vi "Database - Read Entry.vi"(0 "reference in":refnum<class "Database_UUT.lvclass">, 4 "Part Number":string, 5 "error in (no error)":errorcluster) -> (9 "Data Waveform":waveform(dbl), 11 "Property Names":string[](array[string]), 13 "Property Values":variant[](array[variant]), 14 "reference out":refnum<class "Database_UUT.lvclass">, 17 "Channel Name":string, 18 "Part Number OUT":string, 19 "error out":errorcluster)   [LabVIEW 2017, in "Database_UUT.lvclass"]
uses:
  Database_UUT.lvclass
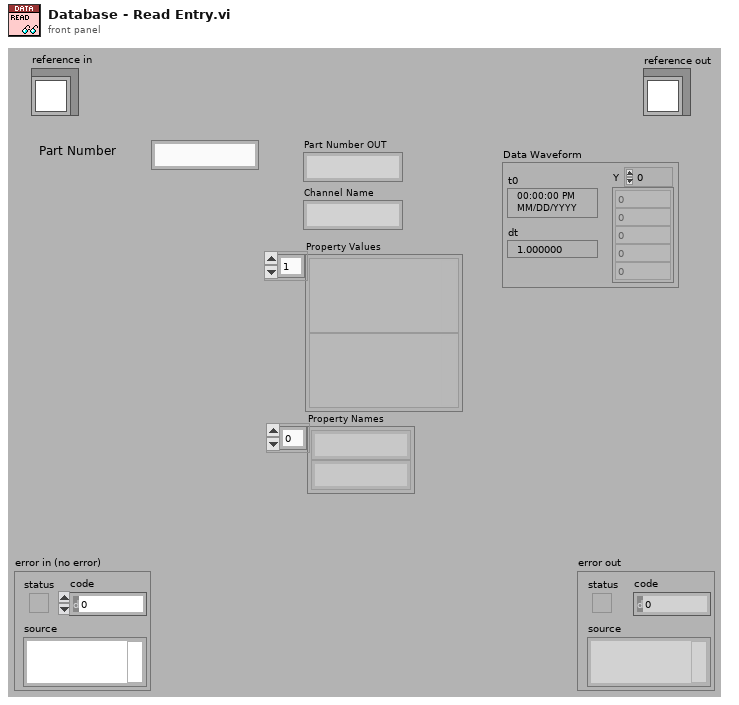
[diagram p1: front panel]
types:
  T1 = enum16{"open", "open or create", "create or replace", "create", "open (read-only)"}
  T2 = typedef "Database_UUT.lvclass/ObjectAttributes.ctl" = cluster{"Filepath to Database":path}
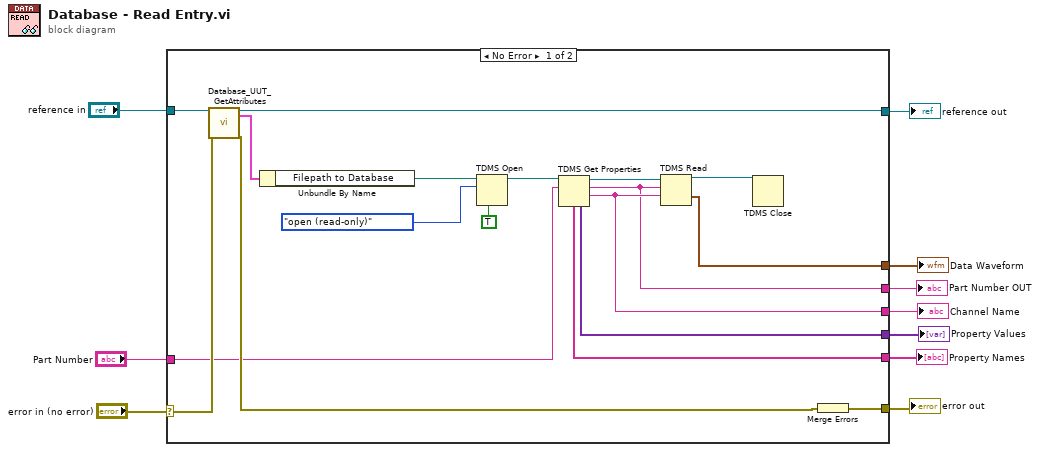
[diagram p0: block diagram]
diagram:
  n1 = case shown="No Error" "error in (no error)" {
    selector: "error in (no error)" -> [w27 w30]
    tunnel: [w23 w30] -> w9
    tunnel: [w25 w29] -> w7
    tunnel: "reference in" -> [w28 w29]
    tunnel: "Part Number" -> [w19 _]
    tunnel: [w12 _] -> w5
    tunnel: [w18 _] -> w4
    tunnel: [w16 _] -> w3
    tunnel: [w14 _] -> w2
    tunnel: [w13 _] -> w1
    frame No Error {
      n2 = call "Database_UUT_GetAttributes.vi"("reference in"=w28, "error in (no error)"=w27) -> ("reference out"=w25:refnum<class "Database_UUT.lvclass">, "Data"=w26:T2, "error out"=w22:errorcluster)  [unwired: 14 in, 1 out]
      n3 = Unbundle By Name(w26) -> ("Filepath to Database"=w21:path)
      n4 = TDMS Open(6:TRUE ("enable asynchronous? (T)"), 10:T1."open (read-only)" ("operation (0:open)"), 11:w21) -> (3:w17:refnum<k34>)  [unwired: 4 in, 1 out]
      n5 = TDMS Get Properties(10:w19, 11:w17) -> (1:w14:string, 2:w12:string, 3:w15:refnum<k34>, 4:w16:variant[], 6:w18:string[])  [unwired: 4 in, 1 out]
      n6 = TDMS Read(0:w15, 5:w12, 7:w14) -> (4:w11:refnum<k34>, 10:w13:waveform(dbl))  [unwired: 5 in, 4 out]
      n7 = TDMS Close(11:w11) -> ()  [unwired: 1 in, 2 out]
      n8 = Merge Errors(w22) -> (w23:errorcluster)
    }
    frame Error {
    }
  }
  "error out" <- w9
  "reference out" <- w7
  "Part Number OUT" <- w5
  "Property Names" <- w4
  "Property Values" <- w3
  "Channel Name" <- w2
  "Data Waveform" <- w1
